vi "get_19572_GB_step_test_time.vi"(8 "error in (no error)":errorcluster, 10 "step":u16=1 min=1 max=99 step=1, 11 "VISA resource in":refnum<visa-resource-name>) -> (0 "error out":errorcluster, 2 "GB total time":string, 3 "VISA resource out":refnum<visa-resource-name>)   [LabVIEW 2015]
doc: "This VI retrieves the test TIME of the selected step and mode."
panel:
  # "Get 19572 GB test time"
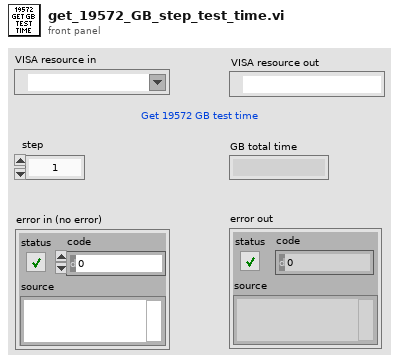
[diagram p1: front panel]
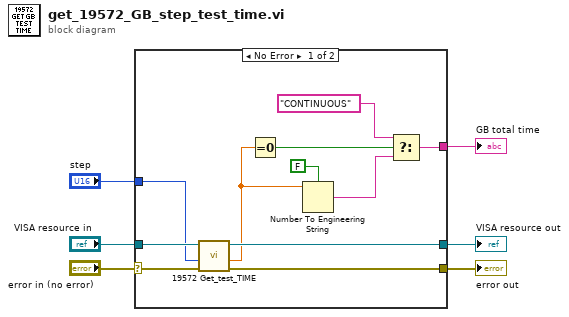
[diagram p0: block diagram]
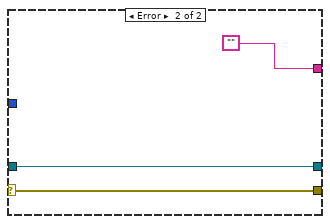
[diagram p2: hidden frame]
diagram:
  n1 = case shown="No Error" "error in (no error)" {
    selector: "error in (no error)" -> [w9 w20]
    tunnel: [w8 w20] -> w6
    tunnel: "VISA resource in" -> [w12 w19]
    tunnel: [w10 w19] -> w4
    tunnel: "step" -> [w11 _]
    tunnel: [w13 ""] -> w2
    frame No Error {
      n2 = call "19572 Get_test_TIME.vi"("error in (no error)"=w9, "Step"=w11, "VISA resource in"=w12) -> ("error out"=w8:errorcluster, "Test TIME"=w7:dbl, "VISA resource out"=w10:refnum<visa-resource-name>)  [unwired: 6 in]
      n3 = Equal To 0?(x=w7) -> (x = 0?=w17:bool)
      n4 = Number To Engineering String(1:FALSE ("use system decimal point (T)"), 4:w7) -> (0:w14:string)  [unwired: 2 in]
      n5 = Select(t="CONTINUOUS", s=w17, f=w14) -> (s? t:f=w13:string)
    }
    frame Error {
    }
  }
  "error out" <- w6
  "VISA resource out" <- w4
  "GB total time" <- w2
